vi "tsdc.vi"() -> ()   [LabVIEW 2010]
uses:
  <vilib>/Instr/_visa.llb/VISA Configure Serial Port (Instr).vi
panel:
  out "value":dbl
  in  "VISA resource name":refnum<visa-resource-name>
  in  "stop":bool
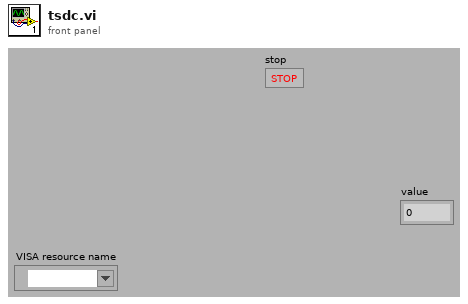
[diagram p1: front panel]
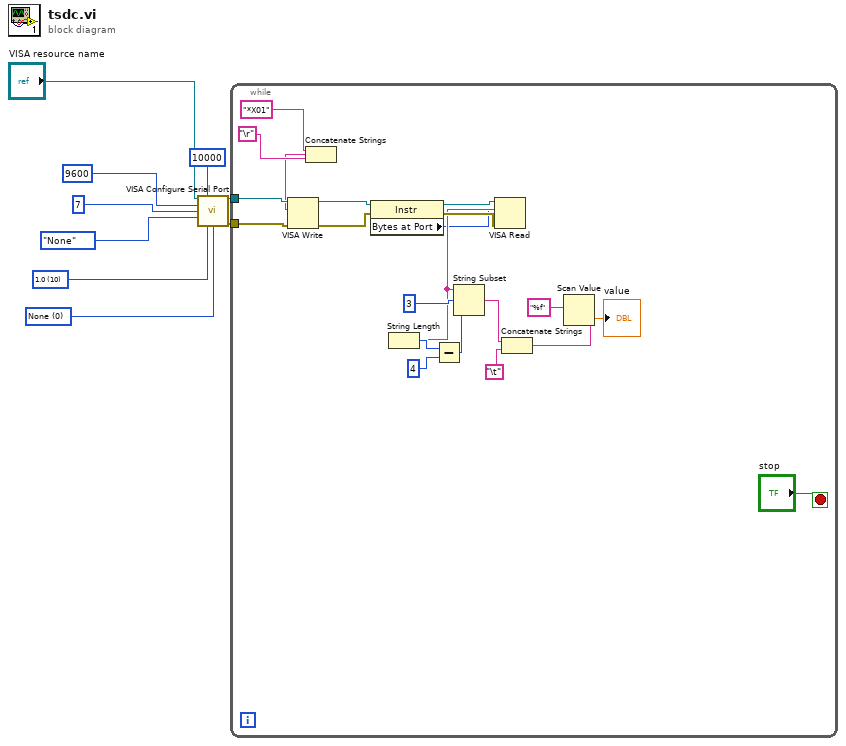
[diagram p0: block diagram]
diagram:
  w3 = u16 0 items=["None", "XON/XOFF", "RTS/CTS", "XON/XOFF & RTS/CTS", "DTR/DSR", "XON/XOFF & DTR/DSR"] ("flow control (0:none)")
  w4 = u16 10 items=["1.0"=10, "1.5"=15, "2.0"=20] ("stop bits (10: 1 bit)")
  n1 = call-poly "VISA Configure Serial Port"("VISA resource name"="VISA resource name", "timeout (10sec)"=u32 10000, "baud rate (9600)"=u32 9600, "data bits (8)"=u16 7, "parity (0:none)"=enum16{"None", "Odd", "Even", "Mark", "Space"}."None", "stop bits (10: 1 bit)"=w4, "flow control (0:none)"=w3) -> ("VISA resource name out"=w9:refnum<visa-resource-name>, "error out"=w2:errorcluster)  [unwired: 7 in]
  n2 = while {
    tunnel: w9 -> [w23]
    tunnel: w2 -> [w21]
    stop <- "stop" stop-if-true
    n3 = Concatenate Strings("*X01", "\r") -> (w22:string)
    n4 = VISA Write(VISA resource name=w23, write buffer=w22, error in (no error)=w21) -> (VISA resource name out=w26:refnum<visa-resource-name>, error out=w29:errorcluster)  [unwired: 1 out]
    n5 = property class="Instr"(reference=w26, error in=w29) -> (reference out=w30:refnum<visa-resource-name>, error out=w28:errorcluster, "Bytes at Port"=w10:u32)
    n6 = VISA Read(VISA resource name=w30, byte count=w10, error in (no error)=w28) -> (read buffer=w14:string)  [unwired: 3 out]
    n7 = String Length(string=w14) -> (length=w18:i32)
    n8 = Subtract(x=w18, y=4) -> (x-y=w13:i32)
    n9 = String Subset(string=w14, offset (0)=3, length (rest)=w13) -> (substring=w12:string)
    n10 = Concatenate Strings(w12, "\t") -> (w16:string)
    n11 = Scan Value(string=w16, format string="%f") -> (value=→"value":dbl)  [unwired: 1 in, 1 out]
  }
